vi "izamin - Min Element Index (CDB).vi"(7 "xInc":i32=1, 11 "x":cdb[](array[numeric])) -> (0 "error":i32, 3 "izamin":i32)   [LabVIEW 2014, in "NI_AALBLAS.lvlib"]
doc: "For real vectors, returns the index of the element that has the minimum absolute value. For complex vectors, the VI returns the index of the element that has the minimum sum of absolute real and imaginary parts."
uses:
  NI_AALBLAS.lvlib
  Fucntion.ctl
  BLAS1 Utility(CDB).vi
panel:
  # "izamin=the index of min(|Re(x)|+|Im(x)|)"
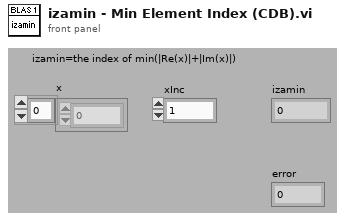
[diagram p1: front panel]
types:
  T1 = typedef "NI_AALBLAS.lvlib/Fucntion.ctl" = u16
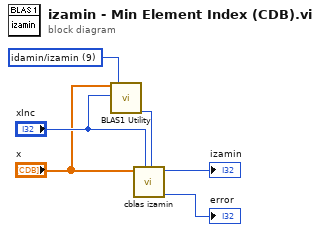
[diagram p0: block diagram]
diagram:
  w1 = T1 9 items=["ddot/zdotu/zdotc", "daxpy/zaxpy", "dnrm2/dznrm2", "dasum/dzasum", "dcopy/zcopy", "dswap/zswap", "drotm", "drot/zdrot", "idamax/izamax", "idamin/izamin", "dgemv/zgemv", "dsymv/zhemv", "dtrmv/ztrmv", "dsyr/zher", "dsyr2/zher2", "dger/zgeru/zgerc", "dtrsv/ztrsv", "dgemm/zgemm", "dsymm/zsymm/zhemm", "dtrmm/ztrmm", "dsyrk/zsyrk/zherk", "dsyr2k/zsyr2k/zher2k", "dtrsm/ztrsm"] ("function")
  n1 = call-poly "BLAS1 Utility.vi"("x"="x", "xInc"="xInc", "function"=w1) -> ("n"=w2:i32)  [unwired: 2 in, 14 out]
  n2 = call "cblas izamin.vi"("n"=w2, "incx"="xInc", "x"="x") -> ("error"=→"error":i32, "izamin"=→"izamin":i32)  [unwired: 7 out]
